vi "calcStiffness.vi"(8 "error in (no error)":errorcluster, 11 "StiffnessMonitor in":refnum<class "StiffnessMonitor.lvclass">) -> (0 "error out":errorcluster, 3 "StiffnessMonitor out":refnum<class "StiffnessMonitor.lvclass">)   [LabVIEW 2013, in "StiffnessMonitor.lvclass"]
uses:
  StiffnessMonitor.lvclass
  Typedefs/ForceDemand.ctl
  StiffnessMonitor.lvclass/StiffnessMonitor.ctl
  Typedefs/FAMTTypedefs.lvlib
panel:
  in  "y":T1=1.0 min=-888.0 max=888.0 format="%.2f"
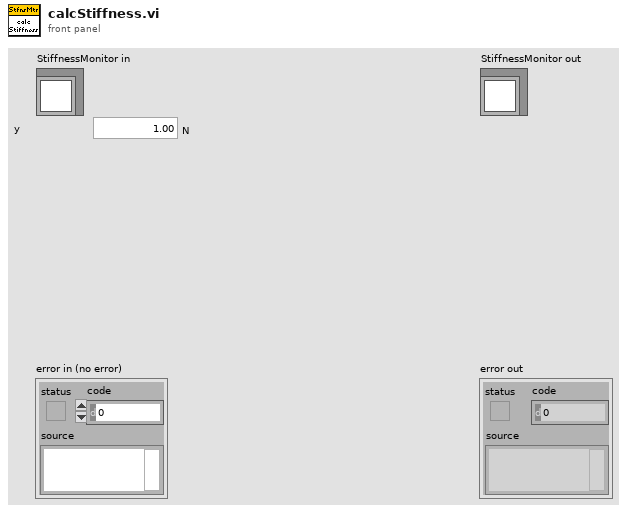
[diagram p1: front panel]
types:
  T1 = typedef "FAMTTypedefs.lvlib/ForceDemand.ctl" = dbl[unit]
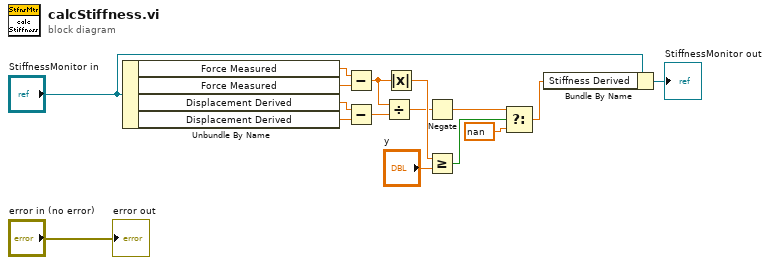
[diagram p0: block diagram]
diagram:
  n1 = Unbundle By Name("StiffnessMonitor in") -> ("Force Measured"=w10:T1, "Force Measured"=w13:T1, "Displacement Derived"=w9:dbl[unit], "Displacement Derived"=w12:dbl[unit])
  n2 = Subtract(x=w10, y=w13) -> (x-y=w8:T1)
  n3 = Subtract(x=w9, y=w12) -> (x-y=w11:dbl[unit])
  n4 = Divide(x=w8, y=w11) -> (x/y=w4:dbl[unit])
  n5 = Absolute Value(x=w8) -> (abs(x)=w7:T1)
  n6 = Negate(x=w4) -> (-x=w1:dbl[unit])
  n7 = Greater Or Equal?(x=w7, y="y") -> (x >= y?=w5:bool)
  n8 = Select(t=w1, s=w5, f=dbl[unit] nan) -> (s? t:f=w2:dbl[unit])
  n9 = Bundle By Name(cluster="StiffnessMonitor in", "Stiffness Derived"=w2) -> (→"StiffnessMonitor out":refnum<class "StiffnessMonitor.lvclass">)
  "error out" <- "error in (no error)"
